vi "FlatToRichni_measurementlink_sessionmanagement_v1_ReserveSessionsRequest.vi"(5 "OutputClusterType":T1, 11 "InputCluster":T3) -> (3 "OutputCluster":T1)   [LabVIEW 2020, in "Measurement Plugin Session Management Client.lvlib"]
uses:
  Measurement Plugin Session Management Client.lvlib
  ni_measurementlink_sessionmanagement_v1_ReserveSessionsRequest_Flat.ctl
  ni_measurementlink_PinMapContext_Flat.ctl
  ni_measurementlink_sessionmanagement_v1_ReserveSessionsRequest.ctl
  ni_measurementlink_PinMapContext.ctl
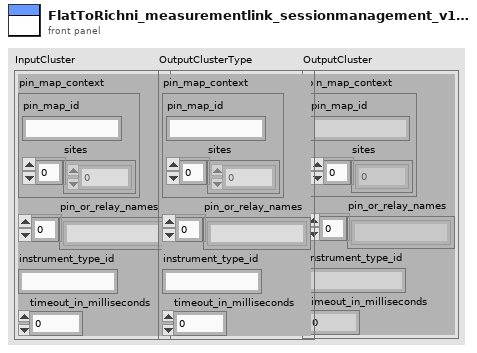
[diagram p1: front panel]
types:
  T1 = typedef "Measurement Plugin Session Management Client.lvlib/ni_measurementlink_sessionmanagement_v1_ReserveSessionsRequest.ctl" = cluster{"pin_map_context":T2, "pin_or_relay_names":string[], "instrument_type_id":string, "timeout_in_milliseconds":i32}
  T2 = typedef "Measurement Plugin Session Management Client.lvlib/ni_measurementlink_PinMapContext.ctl" = cluster{"pin_map_id":string, "sites":i32[]}
  T3 = typedef "Measurement Plugin Session Management Client.lvlib/ni_measurementlink_sessionmanagement_v1_ReserveSessionsRequest_Flat.ctl" = cluster{"pin_map_context":T4, "pin_or_relay_names":string[], "instrument_type_id":string, "timeout_in_milliseconds":i32}
  T4 = typedef "Measurement Plugin Session Management Client.lvlib/ni_measurementlink_PinMapContext_Flat.ctl" = cluster{"pin_map_id":string, "sites":i32[]}
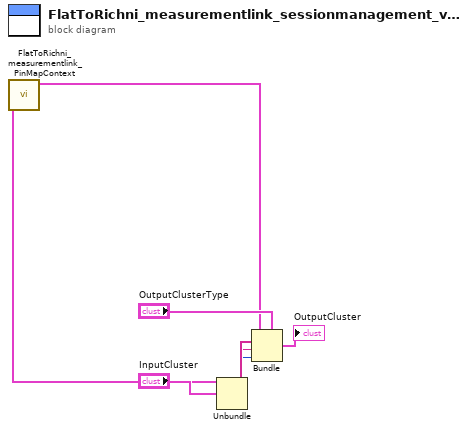
[diagram p0: block diagram]
diagram:
  n1 = Unbundle "Unbundle"("InputCluster") -> ("pin_map_context"=w5:T4, "pin_or_relay_names"=w3:string[], "instrument_type_id"=w2:string, "timeout_in_milliseconds"=w1:i32)
  n2 = call "FlatToRichni_measurementlink_PinMapContext.vi"("InputCluster"=w5) -> ("OutputCluster"=w4:T2)  [unwired: 10 in]
  n3 = Bundle "Bundle"(cluster="OutputClusterType", "pin_map_context"=w4, "pin_or_relay_names"=w3, "instrument_type_id"=w2, "timeout_in_milliseconds"=w1) -> (→"OutputCluster":T1)
